vi "Compare Variants.vi"(8 "error in (no error)":errorcluster, 9 "Variant 2":variant, 10 "Variant 1":variant, 11 "Tolerant Numeric Comparator In":refnum<class "Tolerant Numeric Comparator.lvclass">) -> (0 "error out":errorcluster, 1 "Description":string, 2 "Equal?":bool)   [LabVIEW 2020, in "Tolerant Numeric Comparator.lvclass"]
uses:
  Tolerant Numeric Comparator.lvclass
  Tolerant Numeric Comparator.lvclass/Tolerant Numeric Comparator.ctl
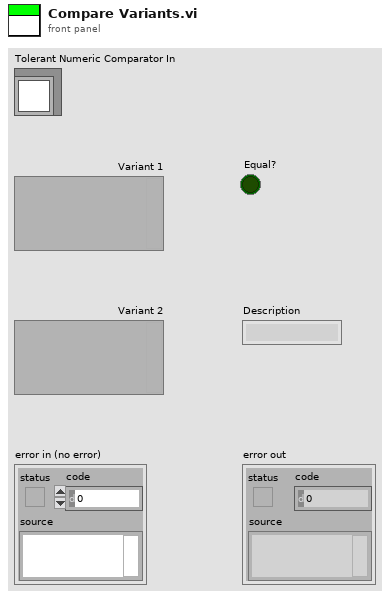
[diagram p1: front panel]
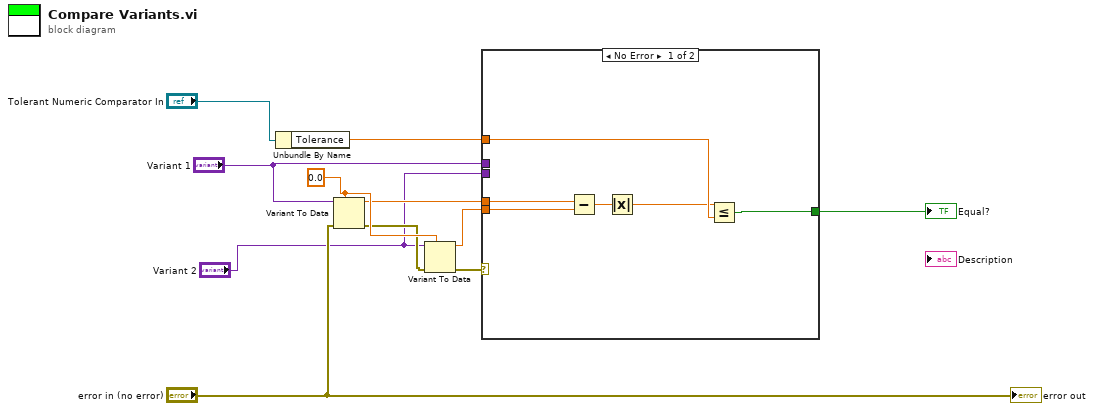
[diagram p0: block diagram]
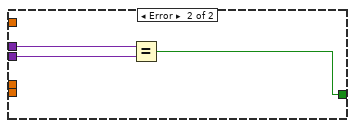
[diagram p2: hidden frame]
diagram:
  w8 = 0.0
  n1 = Unbundle By Name("Tolerant Numeric Comparator In") -> ("Tolerance"=w9:dbl)
  n2 = Variant To Data(error in="error in (no error)", type=w8, Variant="Variant 1") -> (data=w7:dbl, error out=w5:errorcluster)
  n3 = Variant To Data(error in=w5, type=w8, Variant="Variant 2") -> (data=w6:dbl, error out=w3:errorcluster)
  n4 = case shown="No Error" w3 {
    tunnel: [w17 w18] -> w11
    tunnel: w9 -> [w16 _]
    tunnel: w7 -> [w13 _]
    tunnel: w6 -> [w12 _]
    tunnel: "Variant 1" -> [_ w20]
    tunnel: "Variant 2" -> [_ w19]
    frame No Error {
      n5 = Subtract(x=w13, y=w12) -> (x-y=w15:dbl)
      n6 = Absolute Value(x=w15) -> (abs(x)=w14:dbl)
      n7 = Less Or Equal?(x=w14, y=w16) -> (x <= y?=w17:bool)
    }
    frame Error {
      n8 = Equal?(x=w20, y=w19) -> (x = y?=w18:bool)
    }
  }
  "Equal?" <- w11
  "error out" <- "error in (no error)"
